vi "Left_control.vi"(1 "V_TF_L":i32, 5 "클러스터":T1, 7 "Param In":T2, 11 "에러 입력(에러 없음)":errorcluster) -> (4 "queue Out":refnum<queue>, 8 "Param out":T2, 15 "에러 출력":errorcluster)   [LabVIEW 2019]
panel:
  in  "queue In":refnum<queue>
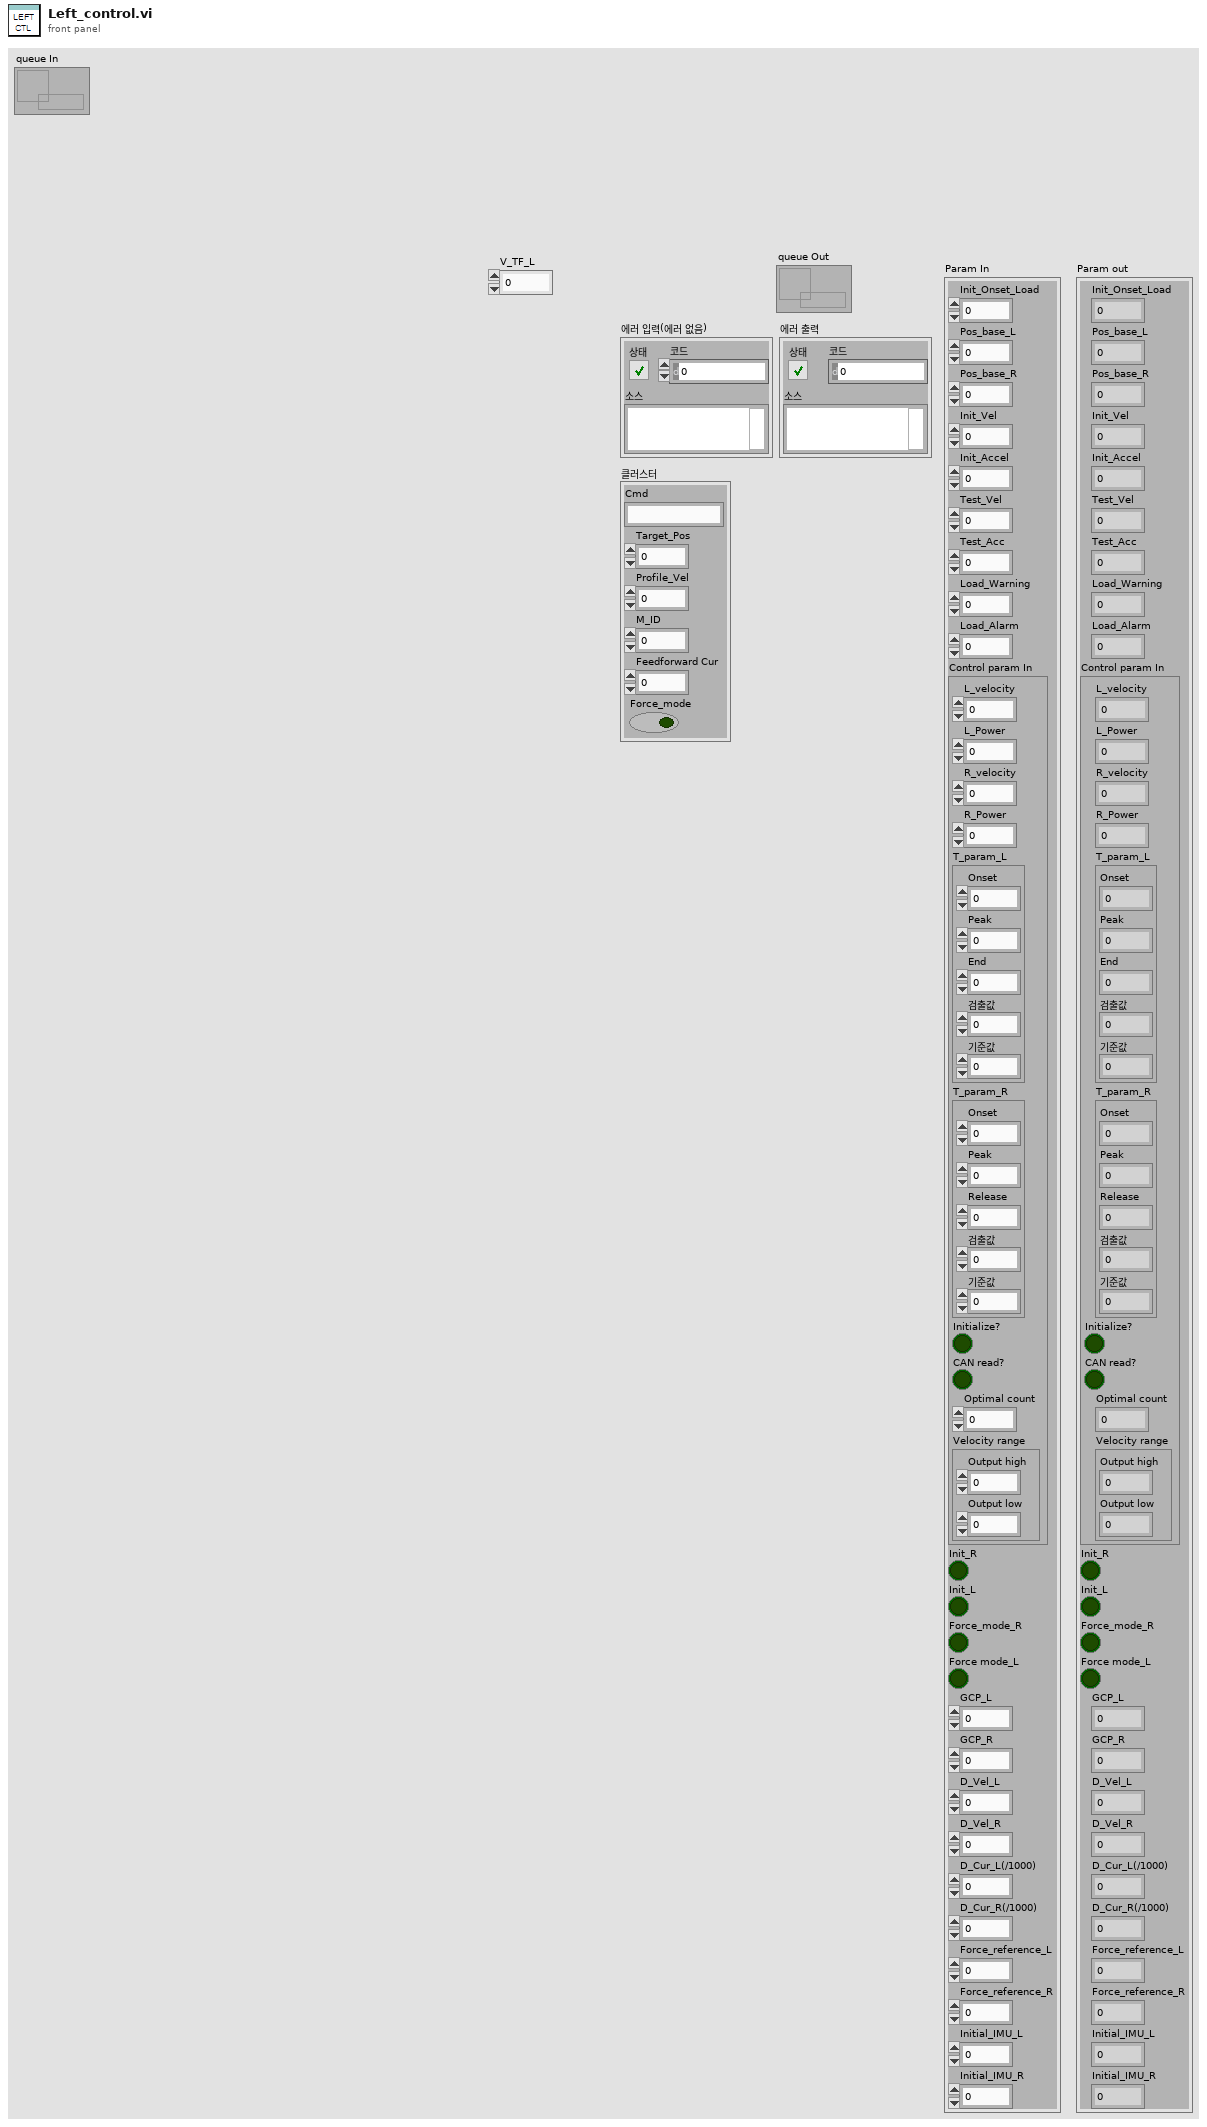
[diagram p1: front panel]
types:
  T1 = cluster{"Cmd":string, "Target_Pos":i32, "Profile_Vel":i32, "M_ID":u8, "Feedforward Cur":i16, "Force_mode":bool}
  T2 = cluster{"Init_Onset_Load":sgl, "Pos_base_L":sgl, "Pos_base_R":sgl, "Init_Vel":i32, "Init_Accel":u32, "Test_Vel":i32, "Test_Acc":u32, "Load_Warning":sgl, "Load_Alarm":sgl, "Control param In":cluster{"L_velocity":u32, "L_Power":sgl, "R_velocity":u32, "R_Power":sgl, "T_param_L":cluster{"Onset":sgl, "Peak":sgl, "End":sgl, "검출값":sgl, "기준값":sgl}, "T_param_R":cluster{"Onset":sgl, "Peak":sgl, "Release":sgl, "검출값":sgl, "기준값":sgl}, "Initialize?":bool, "CAN read?":bool, "Optimal count":i32, "Velocity range":cluster{"Output high":dbl, "Output low":dbl}}, "Init_R":bool, "Init_L":bool, "Force_mode_R":bool, "Force mode_L":bool, "GCP_L":sgl, "GCP_R":sgl, "D_Vel_L":sgl, "D_Vel_R":sgl, "D_Cur_L(/1000)":sgl, "D_Cur_R(/1000)":sgl, "Force_reference_L":sgl, "Force_reference_R":sgl, "Initial_IMU_L":sgl, "Initial_IMU_R":sgl}
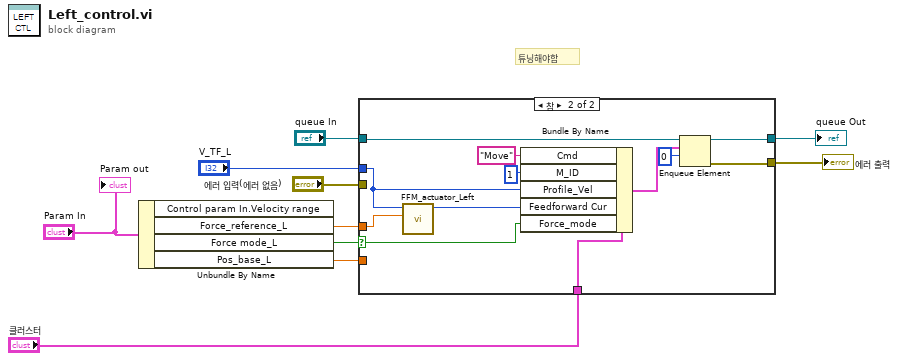
[diagram p0: block diagram]
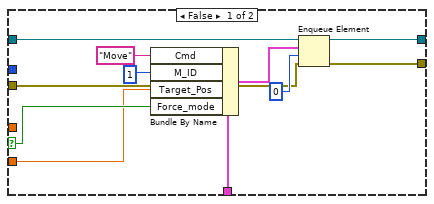
[diagram p2: hidden frame]
diagram:
  # "튜닝해야함"
  n1 = Unbundle By Name("Param In") -> ("Force_reference_L"=w9:sgl, "Force mode_L"=w8:bool, "Pos_base_L"=w10:sgl)  [unwired: 1 out]
  n2 = case shown="참" w8 {
    selector: w8 -> [w19 w24]
    tunnel: w9 -> [_ w33]
    tunnel: w10 -> [w18 _]
    tunnel: "V_TF_L" -> [_ w22]
    tunnel: "클러스터" -> [w15 w25]
    tunnel: "queue In" -> [w14 w28]
    tunnel: "에러 입력(에러 없음)" -> [w13 _]
    tunnel: [w12 w26] -> w3
    tunnel: [w11 w27] -> w4
    frame False {
      n3 = Bundle By Name(cluster=w15, "Cmd"="Move", "M_ID"=u8 1, "Target_Pos"=w18, "Force_mode"=w19) -> (w16:T1)
      n4 = Enqueue Element(queue=w14, element=w16, timeout in ms (-1)=0 ("타임아웃(ms) (-1)"), error in (no error)=w13) -> (queue out=w11:refnum<queue>, error out=w12:errorcluster)  [unwired: 1 out]
    }
    frame True {
      n5 = call "FFM_actuator_Left.vi"("Force_reference_L"=w33, "V_TF_L"=w22) -> ("숫자형"=w23:i16)  [unwired: 9 in]
      n6 = Bundle By Name(cluster=w25, "Cmd"="Move", "M_ID"=u8 1, "Profile_Vel"=w22, "Feedforward Cur"=w23, "Force_mode"=w24) -> (w29:T1)
      n7 = Enqueue Element(queue=w28, element=w29, timeout in ms (-1)=0 ("타임아웃(ms) (-1)")) -> (queue out=w27:refnum<queue>, error out=w26:errorcluster)  [unwired: 1 in, 1 out]
    }
  }
  "에러 출력" <- w3
  "queue Out" <- w4
  "Param out" <- "Param In"
